vi "Set Offset Tuning.vi"(8 "error in (no error)":errorcluster, 10 "Offset Tuning":bool, 11 "RTL-SDR in":refnum<class "RTL-SDR.lvclass">) -> (0 "error out":errorcluster, 1 "function return":i32, 3 "RTL-SDR out":refnum<class "RTL-SDR.lvclass">)   [LabVIEW 2015, in "RTL-SDR.lvclass"]
doc: "Created IvanLis by LabVIEW Portal\nProfile: http://labviewportal.org/memberlist.php?mode=viewprofile&u=987\neMail: IvanLisanov@gMail.com\nTelegram: https://t.me/IvanLis"
uses:
  RTL-SDR.lvclass
  RTL-SDR.lvclass/RTL-SDR.ctl
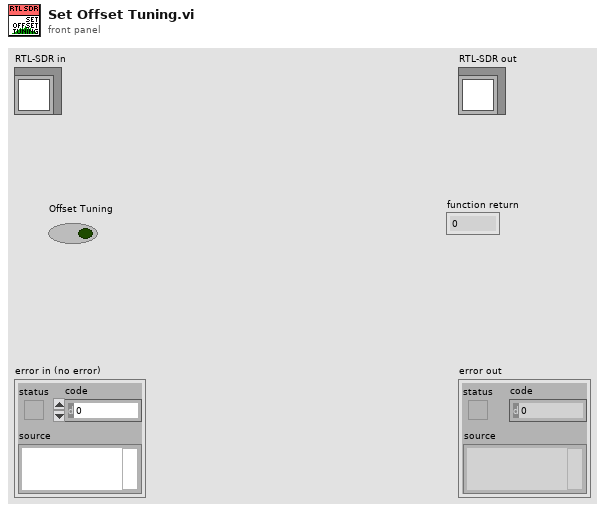
[diagram p1: front panel]
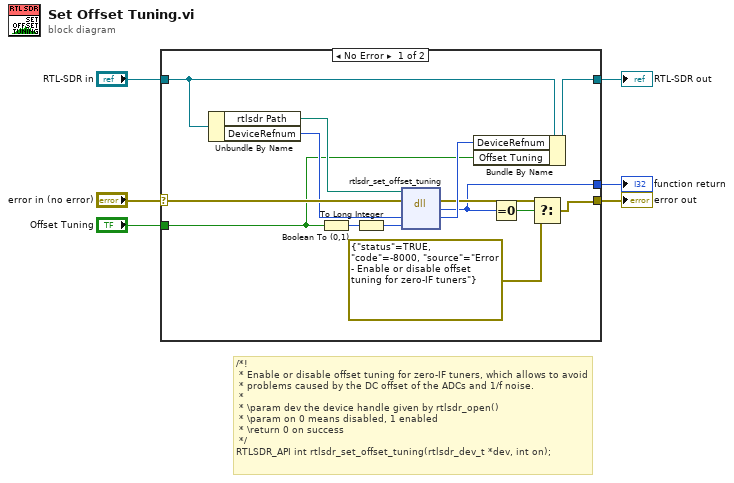
[diagram p0: block diagram]
diagram:
  # "/*!\n * Enable or disable offset tuning for zero-IF tuners, which allows to avoid\n * problems caused by the DC offset of the ADCs and 1/f noise.\n *\n * \\param dev the device handle given by rtlsdr_open()\n * \\param on 0 means disabled, 1 enabled\n * \\return 0 on success\n */\nRTLSDR_API int rtlsdr_set_offset_tuning(rtlsdr_dev_t *dev, int on);"
  n1 = case shown="No Error" "error in (no error)" {
    selector: "error in (no error)" -> [w20 w22]
    tunnel: [w7 w22] -> w5
    tunnel: [w18 w21] -> w3
    tunnel: "RTL-SDR in" -> [w19 w21]
    tunnel: [w8 _] -> w2
    tunnel: "Offset Tuning" -> [w12 _]
    frame No Error {
      n2 = Unbundle By Name(w19) -> ("rtlsdr Path"=w17:path, "DeviceRefnum"=w16:u64)
      n3 = Boolean To (0,1)(Boolean=w12) -> (0, 1=w14:i16)
      n4 = To Long Integer(number=w14) -> (32bit integer=w13:i32)
      n5 = dll-call lib="C:/Users/Ivan/Desktop/D-23-09-24 (RTL-SDR)/Project (Pelleng-SDR)/RTL-SDR Class/dll/rtlsdr.*" fn="rtlsdr_set_offset_tuning"(path in=w17, error in=w20, "DeviceRefnum"=w16, "Offset Tuning"=w13) -> (error out=w9:errorcluster, "return type"=w8:i32, "DeviceRefnum"=w15:u64)  [unwired: 2 in, 1 out]
      n6 = Bundle By Name(cluster=w19, "DeviceRefnum"=w15, "Offset Tuning"=w12) -> (w18:refnum<class "RTL-SDR.lvclass">)
      n7 = Equal To 0?(x=w8) -> (x = 0?=w11:bool)
      n8 = Select(t=w9, s=w11, f=errorcluster {"status"=TRUE, "code"=-8000, "source"="Error - Enable or disable offset tuning for zero-IF tuners"} ("error out")) -> (s? t:f=w7:errorcluster)
    }
    frame Error {
    }
  }
  "error out" <- w5
  "RTL-SDR out" <- w3
  "function return" <- w2
